vi "Write Anything.vi"(7 "Format String (%#_13g)":string="%#_13g", 8 "Error In":errorcluster, 9 "Section Name (Name of \"Anything\")":string, 10 "Anything":variant, 11 "Path (dialog)":path) -> (0 "Error Out":errorcluster, 3 "Path out":path)   [LabVIEW 2020]
doc: "This VI is designed to write any data type to an INI file in human readable form. It will overwrite any data in the specified section of the INI file but leave other sections unchanged.\n\nFreeware from Moore Good Ideas, www.mooregoodideas.com. Do not remove this line."
uses:
  Koop/KObject Class/KObject.lvclass
  <vilib>/Utility/VariantDataType/VariantType.lvlib
  <vilib>/Utility/Data Type/NI_Data Type.lvlib
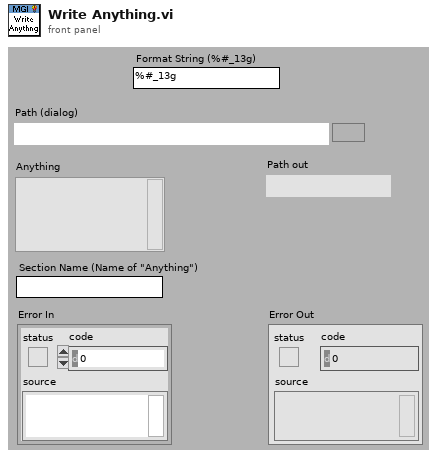
[diagram p1: front panel]
types:
  T1 = typedef "VariantType.lvlib/Type.ctl" = enum8{"Invalid Type", "Void", "I8", "I16", "I32", "I64", "U8", "U16", "U32", "U64", "Single Float", "Double Float", "Extended Float", "Single Complex", "Double Complex", "Extended Complex", "Enum U8", "Enum U16", "Enum U32", "Enum U64", "Single Float With Unit", "Double Float With Unit", "Extended Float With Unit", "Single Complex with Unit", "Double Complex with Unit", "Extended Complex with Unit", "Boolean", "String", "Path", "Picture", "Tag", "Array", "Cluster", "Variant", "LV Variant", "Waveform", "Timestamp", "Digital Waveform", "Digital Data", "ExpressData", "Refnum", "External Data", "VI", "Poly VI", "LabVIEW Class Instance", "Fixed Point"}
  T2 = typedef "NI_Data Type.lvlib/Data Type.ctl" = enum8{"Invalid Type", "Void", "I8", "I16", "I32", "I64", "U8", "U16", "U32", "U64", "Single Float", "Double Float", "Extended Float", "Single Complex", "Double Complex", "Extended Complex", "Enum U8", "Enum U16", "Enum U32", "Enum U64", "Single Float With Unit", "Double Float With Unit", "Extended Float With Unit", "Single Complex with Unit", "Double Complex with Unit", "Extended Complex with Unit", "Boolean", "String", "Path", "Picture", "Tag", "Array", "Cluster", "Variant", "LV Variant", "Waveform", "Timestamp", "Digital Waveform", "Digital Data", "ExpressData", "Refnum", "External Data", "VI", "Poly VI", "LabVIEW Class Instance", "Fixed Point", "Set Collection", "Map Collection"}
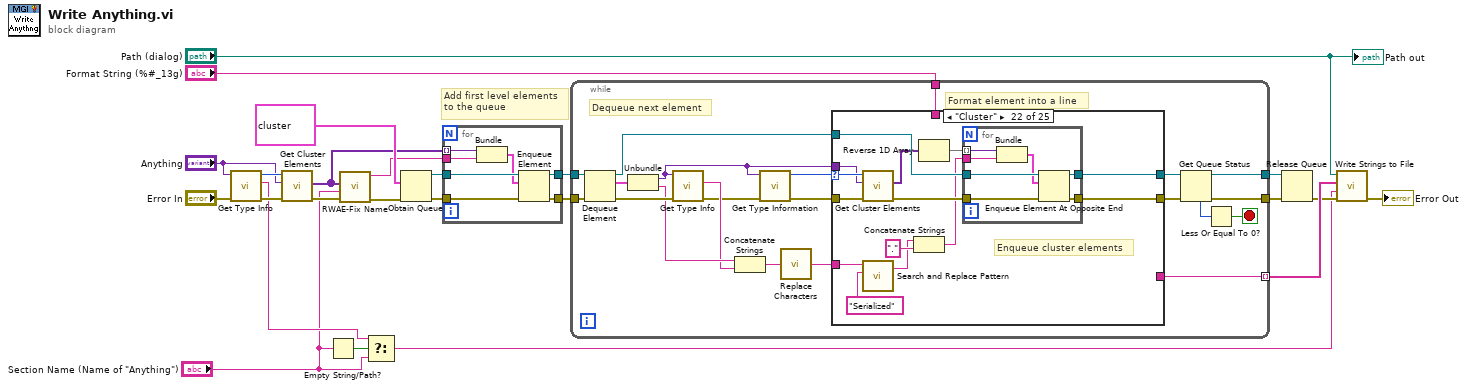
[diagram p0: block diagram]
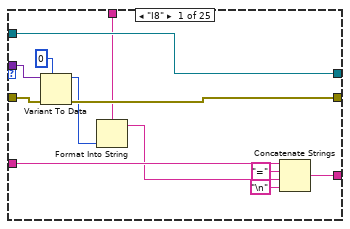
[diagram p2: hidden frame]
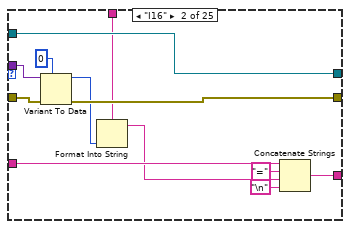
[diagram p3: hidden frame]
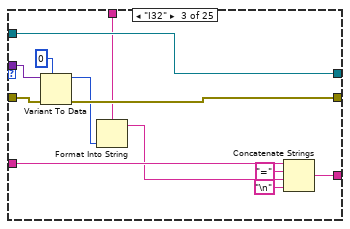
[diagram p4: hidden frame]
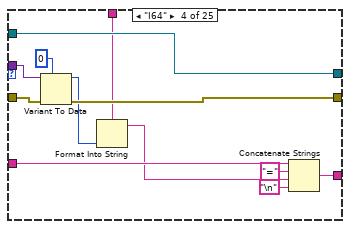
[diagram p5: hidden frame]
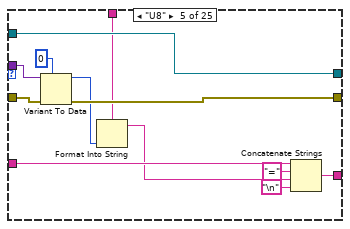
[diagram p6: hidden frame]
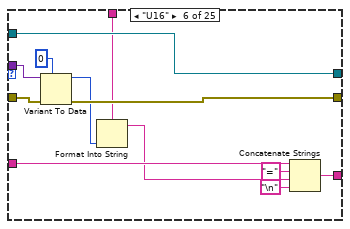
[diagram p7: hidden frame]
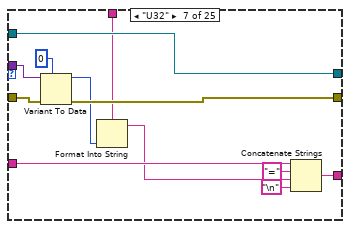
[diagram p8: hidden frame]
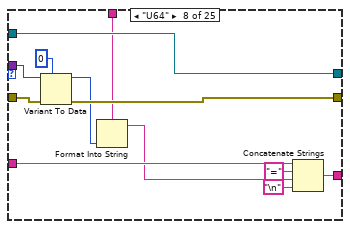
[diagram p9: hidden frame]
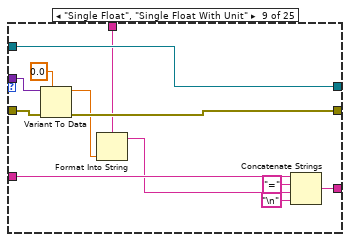
[diagram p10: hidden frame]
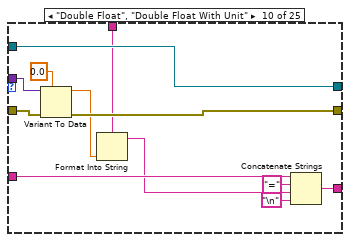
[diagram p11: hidden frame]
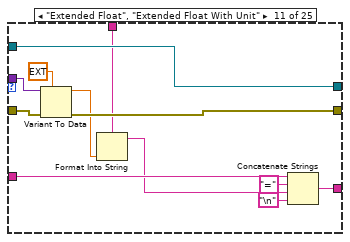
[diagram p12: hidden frame]
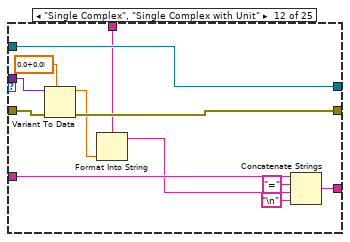
[diagram p13: hidden frame]
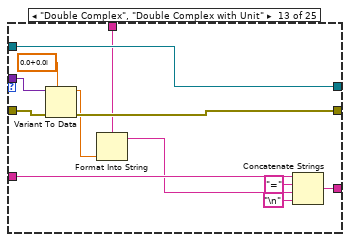
[diagram p14: hidden frame]
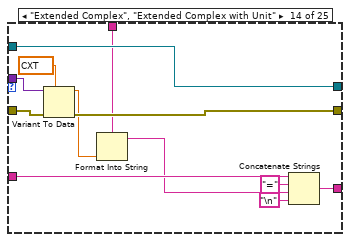
[diagram p15: hidden frame]
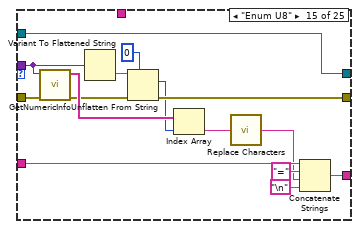
[diagram p16: hidden frame]
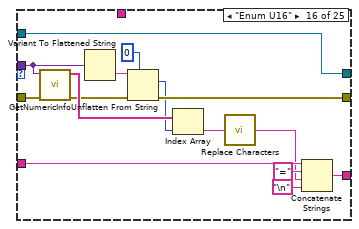
[diagram p17: hidden frame]
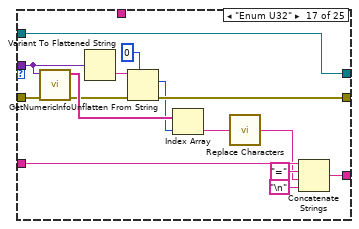
[diagram p18: hidden frame]
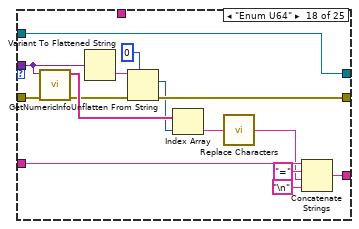
[diagram p19: hidden frame]
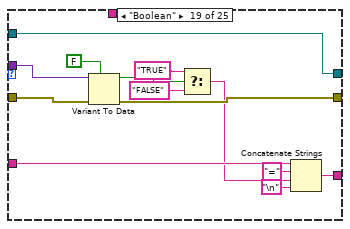
[diagram p20: hidden frame]
diagram:
  # "Add first level elements\nto the queue"
  n1 = call "Get Type Info.vi"("Error In"="Error In", "Variant"="Anything") -> ("Error Out"=w15:errorcluster, "Name"=w9:string, "Type Enum"=w12:T1)  [unwired: 7 in]
  n2 = call "Get Cluster Elements.vi"("Error In"=w15, "Cluster"="Anything", "Type Enum (Cluster)"=w12) -> ("Error Out"=w5:errorcluster, "Cluster Elements"=w2:variant[])  [unwired: 7 in]
  n3 = Empty String/Path?(string/path="Section Name (Name of \"Anything\")") -> (empty?=w10:bool)
  n4 = call "RWAE-Fix Name.vi"("error in (no error)"=w5, "Section Name (Name of \"Anything\")"="Section Name (Name of \"Anything\")", "Cluster Elements in"=w2) -> ("error out"=w1:errorcluster, "Name"=w3:string)  [unwired: 7 in]
  n5 = Select(t=w9, s=w10, f="Section Name (Name of \"Anything\")") -> (s? t:f=w8:string)
  n6 = Obtain Queue(element data type=cluster{"Variant":variant, "Name":string} {"Variant"=variant, "Name"=""}, error in (no error)=w1) -> (queue out=w23:refnum<queue>, error out=w22:errorcluster)  [unwired: 3 in, 1 out]
  n7 = for {
    tunnel: w23 -> [w31]
    tunnel: w22 -> [w30]
    tunnel: [w29] -> w21
    tunnel: [w28] -> w20
    tunnel: w3 -> [w26]
    tunnel: w2 -> [w25] mode=indexing
    n8 = Bundle("Variant"=w25, "Name"=w26) -> (w27:cluster{"Variant":variant, "Name":string})  [unwired: 1 in]
    n9 = Enqueue Element(queue=w31, element=w27, error in (no error)=w30) -> (queue out=w28:refnum<queue>, error out=w29:errorcluster)  [unwired: 1 in, 1 out]
  }
  n10 = while {
    tunnel: w21 -> [w52]
    tunnel: [w49] -> w19
    tunnel: [w40] -> w24 mode=indexing
    tunnel: w20 -> [w50]
    tunnel: [w46] -> w18
    tunnel: "Format String (%#_13g)" -> [w36]
    stop <- w47 stop-if-true
    # "Format element into a line"
    # "Dequeue next element"
    n11 = Dequeue Element(queue=w50, error in (no error)=w52) -> (queue out=w44:refnum<queue>, element=w42:cluster{"Variant":variant, "Name":string}, error out=w51:errorcluster)  [unwired: 1 in, 1 out]
    n12 = Unbundle(w42) -> ("Variant"=w34:variant, "Name"=w41:string)
    n13 = call "Get Type Info.vi"("Error In"=w51, "Variant"=w34) -> ("Error Out"=w33:errorcluster, "Name"=w39:string)  [unwired: 7 in, 1 out]
    n14 = Concatenate Strings(w41, w39) -> (w38:string)
    n15 = call <vilib>:"Get Type Information.vi"("error in (no error)"=w33, "variant"=w34) -> ("error out"=w32:errorcluster, "type"=w35:T2)  [unwired: 5 in, 3 out]
    n16 = call "Replace Characters.vi"("String In"=w38) -> ("String Out"=w37:string)  [unwired: 1 in]
    n17 = case shown="\"Cluster\"" w35 {
      selector: w35 -> [_ _ _ _ _ _ _ _ _ _ _ _ _ _ _ _ _ _ _ _ _ w324 _ _ _]
      tunnel: [w64 w76 w88 w100 w112 w124 w136 w148 w160 w172 w184 w196 w208 w220 w235 w250 w265 w280 w293 w304 w316 w328 w344 w361 w363] -> w45
      tunnel: w44 -> [w64 w76 w88 w100 w112 w124 w136 w148 w160 w172 w184 w196 w208 w220 w235 w250 w265 w280 w293 w304 w316 w329 w348 w361 w363]
      tunnel: [w60 w72 w84 w96 w108 w120 w132 w144 w156 w168 w180 w192 w204 w216 w229 w244 w259 w274 w292 w303 w315 w330 w345 w360 w365] -> w43
      tunnel: w32 -> [w63 w75 w87 w99 w111 w123 w135 w147 w159 w171 w183 w195 w207 w219 w234 w249 w264 w279 w289 w300 w312 w326 w346 w360 w362]
      tunnel: w37 -> [w57 w68 w80 w92 w104 w116 w128 w140 w152 w164 w176 w187 w199 w211 w223 w238 w253 w268 w282 w296 w307 w319 w340 w350 w369]
      tunnel: w34 -> [w62 w74 w86 w98 w110 w122 w134 w146 w158 w170 w182 w194 w206 w218 w232 w247 w262 w277 w290 w301 w313 w323 w347 w359 w367]
      tunnel: [w56 w69 w81 w93 w105 w117 w129 w141 w153 w165 w177 w188 w200 w212 w224 w239 w254 w269 w283 w297 w308 _ w341 w351 _] -> w40
      tunnel: w36 -> [w53 w65 w77 w91 w101 w113 w125 w137 w149 w162 w173 w185 w197 w209 _ _ _ _ _ _ _ _ w338 _ _]
      frame "I8" {
        n18 = Variant To Data(error in=w63, type=i8 0, Variant=w62) -> (data=w55:i8, error out=w60:errorcluster)
        n19 = Format Into String(format string=w53, w55) -> (resulting string=w54:string)  [unwired: 2 in, 1 out]
        n20 = Concatenate Strings(w57, "=" ("string"), w54, "\n") -> (w56:string)
      }
      frame "I16" {
        n21 = Variant To Data(error in=w75, type=i16 0, Variant=w74) -> (data=w66:i16, error out=w72:errorcluster)
        n22 = Format Into String(format string=w65, w66) -> (resulting string=w67:string)  [unwired: 2 in, 1 out]
        n23 = Concatenate Strings(w68, "=" ("string"), w67, "\n") -> (w69:string)
      }
      frame "I32" {
        n24 = Variant To Data(error in=w87, type=0, Variant=w86) -> (data=w79:i32, error out=w84:errorcluster)
        n25 = Format Into String(format string=w77, w79) -> (resulting string=w78:string)  [unwired: 2 in, 1 out]
        n26 = Concatenate Strings(w80, "=" ("string"), w78, "\n") -> (w81:string)
      }
      frame "I64" {
        n27 = Variant To Data(error in=w99, type=i64 0, Variant=w98) -> (data=w90:i64, error out=w96:errorcluster)
        n28 = Format Into String(format string=w91, w90) -> (resulting string=w89:string)  [unwired: 2 in, 1 out]
        n29 = Concatenate Strings(w92, "=" ("string"), w89, "\n") -> (w93:string)
      }
      frame "U8" {
        n30 = Variant To Data(error in=w111, type=u8 0, Variant=w110) -> (data=w103:u8, error out=w108:errorcluster)
        n31 = Format Into String(format string=w101, w103) -> (resulting string=w102:string)  [unwired: 2 in, 1 out]
        n32 = Concatenate Strings(w104, "=" ("string"), w102, "\n") -> (w105:string)
      }
      frame "U16" {
        n33 = Variant To Data(error in=w123, type=u16 0, Variant=w122) -> (data=w115:u16, error out=w120:errorcluster)
        n34 = Format Into String(format string=w113, w115) -> (resulting string=w114:string)  [unwired: 2 in, 1 out]
        n35 = Concatenate Strings(w116, "=" ("string"), w114, "\n") -> (w117:string)
      }
      frame "U32" {
        n36 = Variant To Data(error in=w135, type=u32 0, Variant=w134) -> (data=w127:u32, error out=w132:errorcluster)
        n37 = Format Into String(format string=w125, w127) -> (resulting string=w126:string)  [unwired: 2 in, 1 out]
        n38 = Concatenate Strings(w128, "=" ("string"), w126, "\n") -> (w129:string)
      }
      frame "U64" {
        n39 = Variant To Data(error in=w147, type=u64 0, Variant=w146) -> (data=w139:u64, error out=w144:errorcluster)
        n40 = Format Into String(format string=w137, w139) -> (resulting string=w138:string)  [unwired: 2 in, 1 out]
        n41 = Concatenate Strings(w140, "=" ("string"), w138, "\n") -> (w141:string)
      }
      frame "Single Float", "Single Float With Unit" {
        n42 = Variant To Data(error in=w159, type=sgl 0.0, Variant=w158) -> (data=w151:sgl, error out=w156:errorcluster)
        n43 = Format Into String(format string=w149, w151) -> (resulting string=w150:string)  [unwired: 2 in, 1 out]
        n44 = Concatenate Strings(w152, "=" ("string"), w150, "\n") -> (w153:string)
      }
      frame "Double Float", "Double Float With Unit" {
        n45 = Variant To Data(error in=w171, type=0.0, Variant=w170) -> (data=w163:dbl, error out=w168:errorcluster)
        n46 = Format Into String(format string=w162, w163) -> (resulting string=w161:string)  [unwired: 2 in, 1 out]
        n47 = Concatenate Strings(w164, "=" ("string"), w161, "\n") -> (w165:string)
      }
      frame "Extended Float", "Extended Float With Unit" {
        n48 = Variant To Data(error in=w183, type=ext 0.0, Variant=w182) -> (data=w175:ext, error out=w180:errorcluster)
        n49 = Format Into String(format string=w173, w175) -> (resulting string=w174:string)  [unwired: 2 in, 1 out]
        n50 = Concatenate Strings(w176, "=" ("string"), w174, "\n") -> (w177:string)
      }
      frame "Single Complex", "Single Complex with Unit" {
        n51 = Variant To Data(error in=w195, type=csg 0.0+0.0i, Variant=w194) -> (data=w191:csg, error out=w192:errorcluster)
        n52 = Format Into String(format string=w185, w191) -> (resulting string=w186:string)  [unwired: 2 in, 1 out]
        n53 = Concatenate Strings(w187, "=" ("string"), w186, "\n") -> (w188:string)
      }
      frame "Double Complex", "Double Complex with Unit" {
        n54 = Variant To Data(error in=w207, type=cdb 0.0+0.0i, Variant=w206) -> (data=w203:cdb, error out=w204:errorcluster)
        n55 = Format Into String(format string=w197, w203) -> (resulting string=w198:string)  [unwired: 2 in, 1 out]
        n56 = Concatenate Strings(w199, "=" ("string"), w198, "\n") -> (w200:string)
      }
      frame "Extended Complex", "Extended Complex with Unit" {
        n57 = Variant To Data(error in=w219, type=cxt 0.0+0.0i, Variant=w218) -> (data=w215:cxt, error out=w216:errorcluster)
        n58 = Format Into String(format string=w209, w215) -> (resulting string=w210:string)  [unwired: 2 in, 1 out]
        n59 = Concatenate Strings(w211, "=" ("string"), w210, "\n") -> (w212:string)
      }
      frame "Enum U8" {
        n60 = call <vilib>:"GetNumericInfo.vi"("error in (no error)"=w234, "Variant"=w232) -> ("error out"=w230:errorcluster, "EnumNames"=w233:string[])  [unwired: 6 in, 2 out]
        n61 = Variant To Flattened String(Variant=w232) -> (data string=w231:string)  [unwired: 1 out]
        n62 = Unflatten From String(type=u8 0, binary string=w231, error in (no error)=w230) -> (value=w228:u8, error out=w229:errorcluster)  [unwired: 2 in, 1 out]
        n63 = Index Array(array=w233, index=w228) -> (element=w222:string)
        n64 = call "Replace Characters.vi"("String In"=w222) -> ("String Out"=w221:string)  [unwired: 1 in]
        n65 = Concatenate Strings(w223, "=" ("string"), w221, "\n") -> (w224:string)
      }
      frame "Enum U16" {
        n66 = call <vilib>:"GetNumericInfo.vi"("error in (no error)"=w249, "Variant"=w247) -> ("error out"=w245:errorcluster, "EnumNames"=w248:string[])  [unwired: 6 in, 2 out]
        n67 = Variant To Flattened String(Variant=w247) -> (data string=w246:string)  [unwired: 1 out]
        n68 = Unflatten From String(type=u16 0, binary string=w246, error in (no error)=w245) -> (value=w243:u16, error out=w244:errorcluster)  [unwired: 2 in, 1 out]
        n69 = Index Array(array=w248, index=w243) -> (element=w237:string)
        n70 = call "Replace Characters.vi"("String In"=w237) -> ("String Out"=w236:string)  [unwired: 1 in]
        n71 = Concatenate Strings(w238, "=" ("string"), w236, "\n") -> (w239:string)
      }
      frame "Enum U32" {
        n72 = call <vilib>:"GetNumericInfo.vi"("error in (no error)"=w264, "Variant"=w262) -> ("error out"=w260:errorcluster, "EnumNames"=w263:string[])  [unwired: 6 in, 2 out]
        n73 = Variant To Flattened String(Variant=w262) -> (data string=w261:string)  [unwired: 1 out]
        n74 = Unflatten From String(type=u32 0, binary string=w261, error in (no error)=w260) -> (value=w258:u32, error out=w259:errorcluster)  [unwired: 2 in, 1 out]
        n75 = Index Array(array=w263, index=w258) -> (element=w252:string)
        n76 = call "Replace Characters.vi"("String In"=w252) -> ("String Out"=w251:string)  [unwired: 1 in]
        n77 = Concatenate Strings(w253, "=" ("string"), w251, "\n") -> (w254:string)
      }
      frame "Enum U64" {
        n78 = call <vilib>:"GetNumericInfo.vi"("error in (no error)"=w279, "Variant"=w277) -> ("error out"=w275:errorcluster, "EnumNames"=w278:string[])  [unwired: 6 in, 2 out]
        n79 = Variant To Flattened String(Variant=w277) -> (data string=w276:string)  [unwired: 1 out]
        n80 = Unflatten From String(type=u64 0, binary string=w276, error in (no error)=w275) -> (value=w273:u64, error out=w274:errorcluster)  [unwired: 2 in, 1 out]
        n81 = Index Array(array=w278, index=w273) -> (element=w267:string)
        n82 = call "Replace Characters.vi"("String In"=w267) -> ("String Out"=w266:string)  [unwired: 1 in]
        n83 = Concatenate Strings(w268, "=" ("string"), w266, "\n") -> (w269:string)
      }
      frame "Boolean" {
        n84 = Variant To Data(error in=w289, type=FALSE, Variant=w290) -> (data=w288:bool, error out=w292:errorcluster)
        n85 = Select(t="TRUE", s=w288, f="FALSE") -> (s? t:f=w281:string)
        n86 = Concatenate Strings(w282, "=" ("string"), w281, "\n") -> (w283:string)
      }
      frame "String" {
        n87 = Variant To Data(error in=w300, type="", Variant=w301) -> (data=w295:string, error out=w303:errorcluster)
        n88 = call "Replace Characters.vi"("String In"=w295) -> ("String Out"=w294:string)  [unwired: 1 in]
        n89 = Concatenate Strings(w296, "=" ("string"), w294, "\n") -> (w297:string)
      }
      frame "Path" {
        n90 = Variant To Data(error in=w312, type=path "", Variant=w313) -> (data=w311:path, error out=w315:errorcluster)
        n91 = Path To String(path=w311) -> (string=w306:string)
        n92 = call "Replace Characters.vi"("String In"=w306) -> ("String Out"=w305:string)  [unwired: 1 in]
        n93 = Concatenate Strings(w307, "=" ("string"), w305, "\n") -> (w308:string)
      }
      frame "Cluster" {
        # "Enqueue cluster elements"
        n94 = call "Get Cluster Elements.vi"("Error In"=w326, "Cluster"=w323, "Type Enum (Cluster)"=w324) -> ("Error Out"=w325:errorcluster, "Cluster Elements"=w322:variant[])  [unwired: 7 in]
        n95 = call <vilib>:"Search and Replace Pattern.vi"("string"=w319, "regular expression (\"\")"="Serialized") -> ("result string"=w318:string)  [unwired: 3 in, 1 out]
        n96 = Concatenate Strings(w318, "." ("string")) -> (w320:string)
        n97 = Reverse 1D Array(array=w322) -> (reversed array=w327:variant[])
        n98 = for {
          tunnel: w329 -> [w337]
          tunnel: w325 -> [w336]
          tunnel: [w335] -> w330
          tunnel: [w334] -> w328
          tunnel: w327 -> [w332] mode=indexing
          tunnel: w320 -> [w331]
          n99 = Bundle("Variant"=w332, w331) -> (w333:cluster{"Variant":variant, string})  [unwired: 1 in]
          n100 = Enqueue Element At Opposite End(queue=w337, element=w333, error in (no error)=w336) -> (queue out=w334:refnum<queue>, error out=w335:errorcluster)  [unwired: 1 in, 1 out]
        }
      }
      frame "Array" {
        n101 = call "Process Array Elements.vi"("Format String (%#0.15f)"=w338, "Error In"=w346, "Name In"=w340, "Array Variant"=w347, "Queue In"=w348) -> ("Error Out"=w345:errorcluster, "Data Out"=w339:string, "Queue Out"=w344:refnum<queue>)  [unwired: 4 in]
        n102 = Concatenate Strings(w340, "=" ("string"), w339, "\n") -> (w341:string)
      }
      frame Default {
        n103 = Variant To Flattened String(Variant=w359) -> (data string=w354:string)  [unwired: 1 out]
        n104 = String To Byte Array(string=w354) -> (unsigned byte array=w358:u8[])
        n105 = Number To Hexadecimal String(1:i16 2 ("width (-)"), 2:w358) -> (0:w357:string[])
        n106 = Concatenate Strings("0x", w357) -> (w349:string)
        n107 = Concatenate Strings(w350, "=" ("string"), w349, "\n") -> (w351:string)
      }
      frame "LabVIEW Class Instance" {
        n108 = Variant To Data(error in=w362, type=refnum<class "KObject.lvclass"> refnum ("KObject"), Variant=w367) -> (data=w366:refnum<class "KObject.lvclass">, error out=w364:errorcluster)
        n109 = case shown="No Error" w364 {
          selector: w364 -> [w373 _]
          tunnel: w369 -> [w376 _]
          tunnel: w366 -> [w375 _]
          tunnel: [w374 w381] -> w365
          tunnel: w363 -> [w372 _]
          tunnel: w362 -> [_ w381]
          frame No Error {
            n110 = call-dynamic "To Variant.vi"("KObject in"=w375, "error in (no error)"=w373) -> ("Array"=w371:variant[], "error out"=w374:errorcluster)  [unwired: 11 in, 1 out]
            n111 = Reverse 1D Array(array=w371) -> (reversed array=w370:variant[])
            n112 = for {
              tunnel: w376 -> [w380]
              tunnel: w372 -> [w379]
              tunnel: w370 -> [w377] mode=indexing
              n113 = Bundle("Variant"=w377, "String Out"=w380) -> (w378:cluster{"Variant":variant, "String Out":string})  [unwired: 1 in]
              n114 = Enqueue Element At Opposite End(queue=w379, element=w378) -> ()  [unwired: 2 in, 3 out]
            }
          }
          frame Error {
          }
        }
      }
    }
    n115 = Get Queue Status(queue=w45, error in (no error)=w43) -> (queue out=w46:refnum<queue>, error out=w49:errorcluster, # elements in queue=w48:i32)  [unwired: 1 in, 5 out]
    n116 = Less Or Equal To 0?(x=w48) -> (x <= 0?=w47:bool)
  }
  n117 = Release Queue(queue=w18, error in (no error)=w19) -> (error out=w13:errorcluster)  [unwired: 1 in, 2 out]
  n118 = call "Write Strings to File.vi"("Error In"=w13, "Section Name"=w8, "Array of Strings"=w24, "Path"="Path (dialog)") -> ("Error Out"=→"Error Out":errorcluster)  [unwired: 7 in]
  "Path out" <- "Path (dialog)"
